vi "Glob_setting.vi"() -> ()   [LabVIEW 2019]
uses:
  Durability/Breakdown-Spec.ctl
  Durability/Capacitor/cap_config.ctl
  Durability/Capacitor/Judge_RC.ctl
  Durability/common/result.ctl
panel:
  in  "result":T1=enum."Completion"
  in  "6.3.9 OFF":dbl
  in  "6.3.9 ON":dbl
  in  "6.3.9 시간":dbl
  in  "6.3.8 작동":dbl
  in  "6.3.8 시간":dbl
  in  "6.3.6 작동 2":dbl
  in  "6.3.6 미작동":dbl
  in  "6.3.6 작동 1":dbl
  in  "6.3.4 미작동":dbl
  in  "6.3.4 작동":dbl
  in  "6.3.3 미작동":dbl
  in  "6.3.3 작동":dbl
  in  "6.3.2 미작동":dbl
  in  "6.3.2 작동":dbl
  in  "Breakdown-Spec":T2={"제어단 단선 Irms[mA](이하)"=5.0, "제어단 특성 전류 Irms[mA] Max"=50.0, "제어단 특성 전류 Irms[mA] Min"=10.0, "출력단 단선 Irms[mA](이하)"=5.0, "출력단 특성 전류 Irms[mA]  Max"=3700.0, "출력단 특성전류 Irms[mA]  Min"=1000.0, "온도[degree]"=0.0} {"출력단 특성전류 Irms[mA]  Min" format="%#.2f"; "출력단 특성 전류 Irms[mA]  Max" format="%#.2f"; "출력단 단선 Irms[mA](이하)" format="%#.2f"; "제어단 특성 전류 Irms[mA] Min" format="%#.2f"; "제어단 특성 전류 Irms[mA] Max" format="%#.2f"; "제어단 단선 Irms[mA](이하)" format="%#.2f"}
  in  "Testconfig":T3={"Test Mode"=enum."6.3.2 저온 작동/방치 시험", "ON time[ms]"=200.0, "OFF time[ms]"=500.0, "1. 작동시간[분]"=10000.0, "2. 미작동시간[분]"=10000.0, "3. 작동시간[분]"=10000.0, "level[V]"=12.0, "duty"=20.0, "Freq"=1.0, "Voltage+[V]"=20.0, "Voltage-[V]"=-20.0, "Current+[A]"=5.0, "Current-[A]"=-5.0, "출력전압[V]"=200.0, "출력전류[A]"=10.0, "OVP Level"=0.0, "OCP Level"=0.0, "Time Div"=2, "Record Len"=5, "방전 기준[V]"=0.0, "Repeate (Each Ch)"=3, "Cycle[N]"=1, "ON/OFF 회 수[N]"=10000.0, "TrigPos[%]"=0.0, "시험시간[분]"=1.0} {"시험시간[분]" min=1.0; "ON/OFF 회 수[N]" min=1.0; "3. 작동시간[분]" min=1.0; "2. 미작동시간[분]" min=1.0; "1. 작동시간[분]" min=1.0; "Time Div" items=["10m", "20ms", "50ms", "100ms", "200ms", "500ms", "1s", "2s", "5s", "10s", "20s", "30s", "1min", "2min", "5min"]; "OFF time[ms]" min=10000.0 max=1000000.0; "Current-[A]" min=-20.0 max=20.0 step=0.001; "Voltage-[V]" min=-115.0 max=115.0 step=0.01; "Current+[A]" min=0.0 max=60.0 step=0.01; "Voltage+[V]" min=0.0 max=120.0 step=0.1; "OCP Level" format="%#_13g"; "OVP Level" format="%#_13g"; "Record Len" items=["10k", "25k", "50k", "100k", "250k", "500k", "1M", "2.5M", "5M", "10M", "25M", "50M", "100M", "250M", "500M", "1G", "2G", "4G", "5G", "10G", "20G", "50G"]; "ON time[ms]" min=50.0 max=2000000.0}
  in  "Test Judgement":T4={"전압 63%[mS] Min"=25.5, "전압 98%[mS] Min"=140.0, "전류 37%[mS] Min"=25.5, "접촉저항[mOhm] Min"=1.0, "출력전류 Irms[mA] Min"=1500.0, "전압 63%[mS] Max"=5.0, "전압 98%[mS] Max"=5.0, "전류 37%[mS] Max"=5.0, "접촉저항[mOhm] Max"=0.5, "출력전류 Irms[mA] Max"=500.0}
  # "제어단"
  # "출력단"
  # "온도기준"
  # "제어단 전압"
  # "출력단 전원"
  # "DL950"
  # "Discharge"
  # "Test Cycle"
  # "작동 설정"
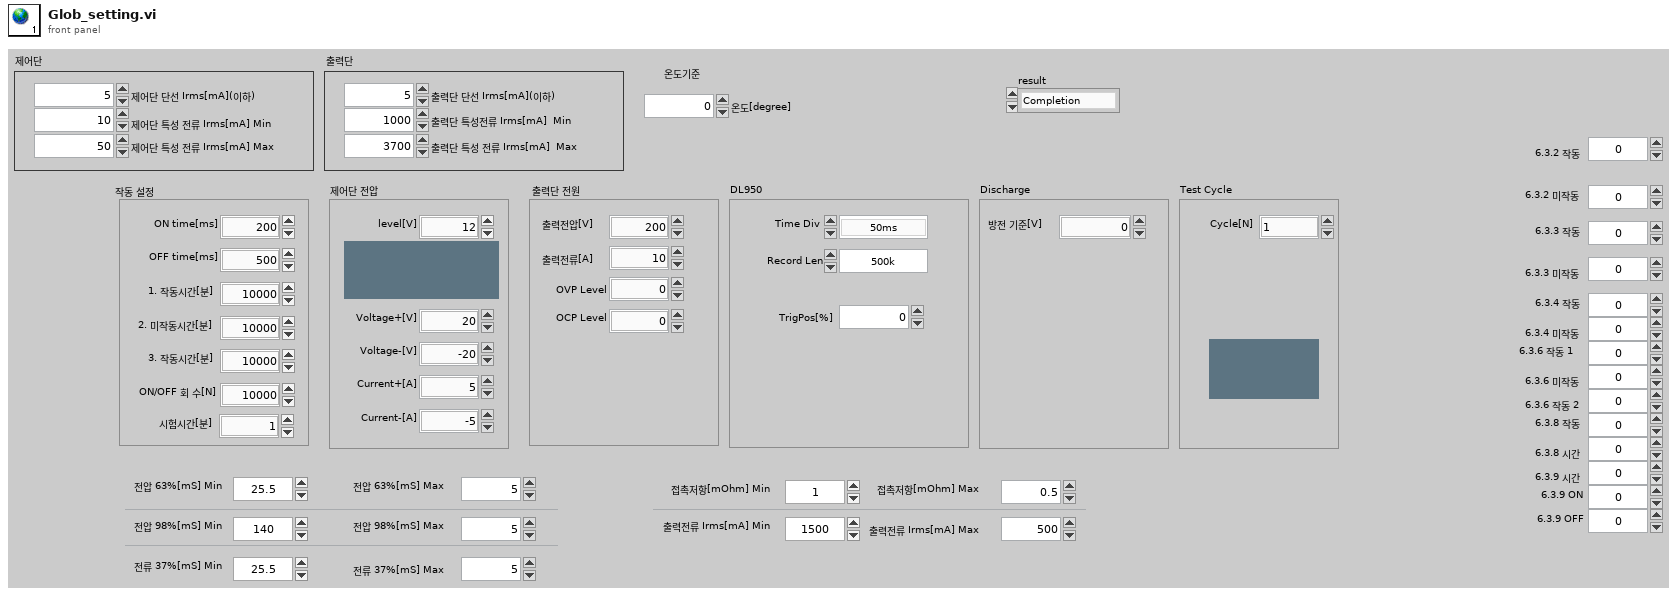
[diagram p1: front panel]
types:
  T1 = typedef "result.ctl" = enum16{"Init", "OK", "NG", "Shutdown", "Testing", "Completion", "Device Error", "Start", "작동", "미작동", "작동 대기", "작동 1"}
  T2 = typedef "Breakdown-Spec.ctl" = cluster{"제어단 단선 Irms[mA](이하)":dbl, "제어단 특성 전류 Irms[mA] Max":dbl, "제어단 특성 전류 Irms[mA] Min":dbl, "출력단 단선 Irms[mA](이하)":dbl, "출력단 특성 전류 Irms[mA]  Max":dbl, "출력단 특성전류 Irms[mA]  Min":dbl, "온도[degree]":dbl}
  T3 = typedef "cap_config.ctl" = cluster{"Test Mode":enum32{"6.3.2 저온 작동/방치 시험", "6.3.3 고온 작동/방치 시험", "6.3.4 온도 싸이클 시험", "6.3.6 온습도 싸이클 시험", "6.3.8 결로 시험", "6.3.9 빙결 시험"}, "ON time[ms]":dbl, "OFF time[ms]":dbl, "1. 작동시간[분]":dbl, "2. 미작동시간[분]":dbl, "3. 작동시간[분]":dbl, "level[V]":dbl, "duty":dbl, "Freq":dbl, "Voltage+[V]":dbl, "Voltage-[V]":dbl, "Current+[A]":dbl, "Current-[A]":dbl, "출력전압[V]":dbl, "출력전류[A]":dbl, "OVP Level":dbl, "OCP Level":dbl, "Time Div":u16, "Record Len":i32, "방전 기준[V]":dbl, "Repeate (Each Ch)":u32, "Cycle[N]":u32, "ON/OFF 회 수[N]":dbl, "TrigPos[%]":dbl, "시험시간[분]":dbl}
  T4 = typedef "Judge_RC.ctl" = cluster{"전압 63%[mS] Min":dbl, "전압 98%[mS] Min":dbl, "전류 37%[mS] Min":dbl, "접촉저항[mOhm] Min":dbl, "출력전류 Irms[mA] Min":dbl, "전압 63%[mS] Max":dbl, "전압 98%[mS] Max":dbl, "전류 37%[mS] Max":dbl, "접촉저항[mOhm] Max":dbl, "출력전류 Irms[mA] Max":dbl}
diagram:
